vi "lab 5-1.vi"() -> ()   [LabVIEW 2021]
panel:
  out "measurement Rs":dbl[](array[numeric])
  out "measurement Ls":dbl[](array[numeric])
  out "relative uncartainty value (%)":dbl
  out "absulate uncartainty":dbl
  out "experimental waste":dbl
  out "best estimated measurement":dbl
  out "sum":dbl
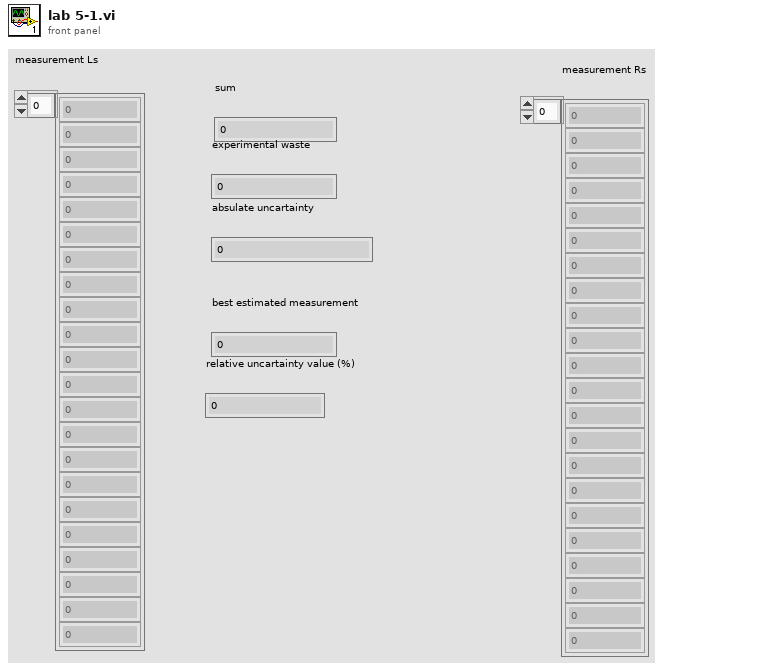
[diagram p1: front panel]
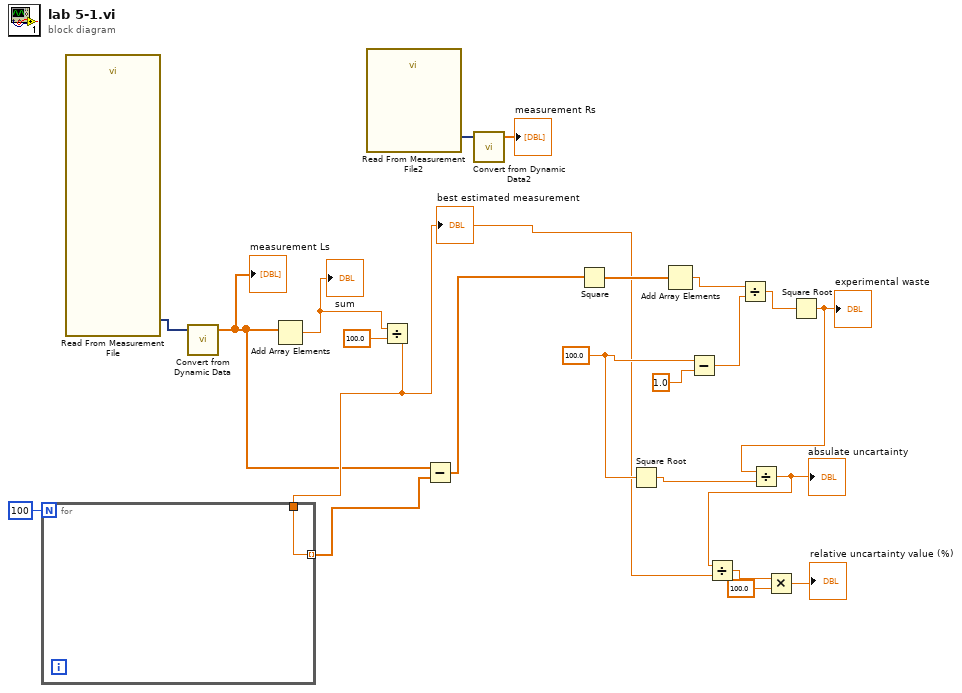
[diagram p0: block diagram]
diagram:
  w12 = 100.0 ("x")
  n1 = call "Read From Measurement File"() -> ("Signals"=w4:dynamicdata)  [unwired: 6 in, 5 out]
  n2 = call "Convert from Dynamic Data"("Dynamic Data Type"=w4) -> ("Array"=w3:dbl[])  [unwired: 3 in]
  "measurement Ls" <- w3
  n3 = Add Array Elements(numeric array=w3) -> (sum=w22:dbl)
  "sum" <- w22
  n4 = call "Read From Measurement File2"() -> ("Signals"=w2:dynamicdata)  [unwired: 6 in, 5 out]
  n5 = Divide(x=w22, y=100.0) -> (x/y=w8:dbl)
  "best estimated measurement" <- w8
  n6 = for {
    N: 100 -> [_]
    tunnel: w8 -> [w23]
    tunnel: [w23] -> w19 mode=indexing
  }
  n7 = Subtract(x=w3, y=w19) -> (x-y=w18:dbl[])
  n8 = call "Convert from Dynamic Data2"("Dynamic Data Type"=w2) -> ("Array"=→"measurement Rs":dbl[])  [unwired: 3 in]
  n9 = Square(x=w18) -> (x^2=w17:dbl[])
  n10 = Square Root(x=w12) -> (sqrt(x)=w10:dbl)
  n11 = Add Array Elements(numeric array=w17) -> (sum=w15:dbl)
  n12 = Subtract(x=w12, y=1.0) -> (x-y=w14:dbl)
  n13 = Divide(x=w15, y=w14) -> (x/y=w13:dbl)
  n14 = Square Root(x=w13) -> (sqrt(x)=w11:dbl)
  "experimental waste" <- w11
  n15 = Divide(x=w11, y=w10) -> (x/y=w9:dbl)
  "absulate uncartainty" <- w9
  n16 = Divide(x=w9, y=w8) -> (x/y=w7:dbl)
  n17 = Multiply(x=w7, y=100.0) -> (x*y=→"relative uncartainty value (%)":dbl)
